vi "Create Coverage Report - Always 100 Lines.vi"() -> ()   [LabVIEW 2017, in "Cobertura.Tests.lvlib"]
uses:
  Cobertura.Tests.lvlib
  Fake Code Inspector/Fake Code Inspector.lvclass
  C:/Users/pasca/Projects/Home/lvunit/Cobertura/Code Inspector Base/Code Inspector Base.lvclass
  Cobertura/Coverage/Coverage.lvclass/Coverage.ctl
  Cobertura/Package/Package.lvclass/Package.ctl
  Cobertura/Class/Class.lvclass/Class.ctl
  Cobertura/Method/Method.lvclass/Method.ctl
  Cobertura/Coverage/Read Packages.vi
  Cobertura/Package/Read Classes.vi
  Cobertura/Class/Read Methods.vi
  Cobertura/Method/Read Lines.vi
  Fake Project Inspector/Fake Project Inspector.lvclass
  C:/Users/pasca/Projects/Home/lvunit/Cobertura/Project Inspector Base/Project Inspector Base.lvclass
  Fake Code Coverage/Fake Code Coverage.lvclass
  C:/Users/pasca/Projects/Home/lvunit/CodeCoverage/CodeCoverage.lvclass
  Cobertura/Package/Package.lvclass
  Cobertura/Class/Class.lvclass
  Cobertura/Method/Method.lvclass
  Cobertura/Line/Line.lvclass
  Cobertura/Cobertura.lvlib
  Cobertura/Coverage/Coverage.lvclass
  <vilib>/PNR/Transparent Assertions/Transparent Assertions/Transparent Assertions.lvlib
panel:
  out "error out":errorcluster
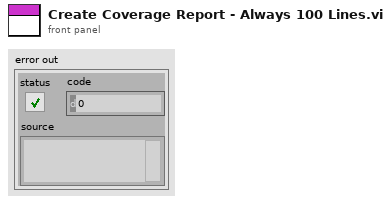
[diagram p1: front panel]
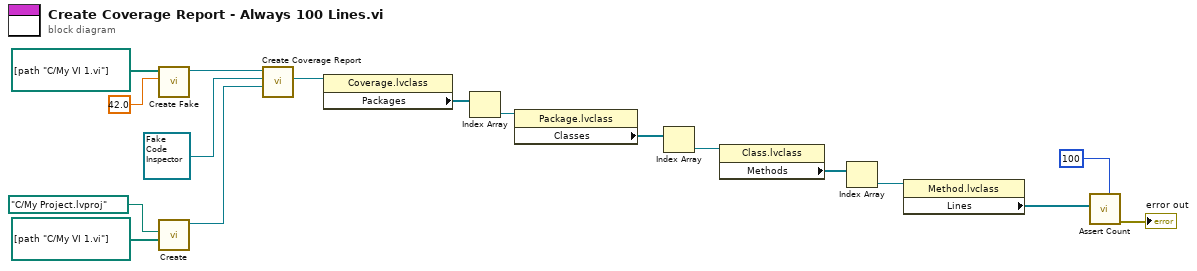
[diagram p0: block diagram]
diagram:
  n1 = call "Create Fake.vi"("Coverage Percentage"=42.0, "All VIs Measured"=path[] [path "C:/My VI 1.vi"] ("Item Paths")) -> ("Fake Code Coverage"=w5:refnum<class "Fake Code Coverage.lvclass">)  [unwired: 8 in, 1 out]
  n2 = call "Create.vi"("Item Paths"=path[] [path "C:/My VI 1.vi"], "Path"=path "C:/My Project.lvproj") -> ("Fake Project Inspector"=w14:refnum<class "Fake Project Inspector.lvclass">)  [unwired: 8 in, 1 out]
  n3 = call "Create Coverage Report.vi"("Project Inspector"=w14, "Code Inspector"=refnum<class "Fake Code Inspector.lvclass"> refnum, "CodeCoverage in"=w5) -> ("Coverage"=w17:refnum<class "Coverage.lvclass">)  [unwired: 7 in, 1 out]
  n4 = property class="Coverage.lvclass"(reference=w17) -> ("Packages"=w15:refnum<class "Package.lvclass">[])  [unwired: 1 in, 2 out]
  n5 = Index Array(array=w15) -> (element=w12:refnum<class "Package.lvclass">)  [unwired: 1 in]
  n6 = property class="Package.lvclass"(reference=w12) -> ("Classes"=w11:refnum<class "Class.lvclass">[])  [unwired: 1 in, 2 out]
  n7 = Index Array(array=w11) -> (element=w9:refnum<class "Class.lvclass">)  [unwired: 1 in]
  n8 = property class="Class.lvclass"(reference=w9) -> ("Methods"=w8:refnum<class "Method.lvclass">[])  [unwired: 1 in, 2 out]
  n9 = Index Array(array=w8) -> (element=w7:refnum<class "Method.lvclass">)  [unwired: 1 in]
  n10 = property class="Method.lvclass"(reference=w7) -> ("Lines"=w6:refnum<class "Line.lvclass">[])  [unwired: 1 in, 2 out]
  n11 = call <vilib>:"Assert Count.vi"("Expected"=100 ("Branch Rate"), "Haystack"=w6) -> ("error out"=→"error out":errorcluster)  [unwired: 9 in]
